vi "DB_CONECTION_PATH.vi"() -> (3 "Conection path":path)   [LabVIEW 2019, in "DB_VENDING MACHINE.lvlib"]
doc: "Aquí se genera la ruta en la que se encuentra nuestro archivo"
uses:
  DB_VENDING MACHINE.lvlib
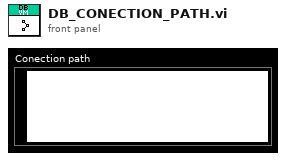
[diagram p1: front panel]
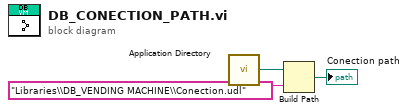
[diagram p0: block diagram]
diagram:
  n1 = call <vilib>:"Application Directory.vi"() -> ("Application Directory"=w3:path)
  n2 = Build Path(base path=w3, name or relative path="Libraries\\DB_VENDING MACHINE\\Conection.udl") -> (appended path=→"Conection path":path)
